vi "Start Node Drag.vi"(0 "FSM in":refnum<class "FSM.Graph.lvclass">, 5 "Node index":i32, 9 "Grid size":dbl, 11 "error in (no error)":errorcluster) -> (4 "FSM out":refnum<class "FSM.Graph.lvclass">, 8 "dragged nodes":string[](array[string]), 15 "error out":errorcluster)   [LabVIEW 2015, in "FSM.Graph.lvclass"]
uses:
  FSM.Graph.lvclass
  FSM.Graph.lvclass/FSM.Graph.ctl
  FSM.Node/FSM.Node.lvclass/FSM.Node.ctl
  FSM.Node/Read Name.vi
  FSM.Node/Read selected.vi
  FSM.Node/FSM.Node.lvclass
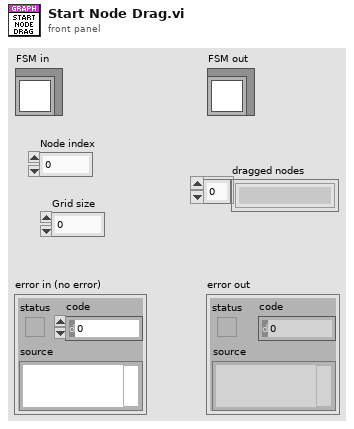
[diagram p1: front panel]
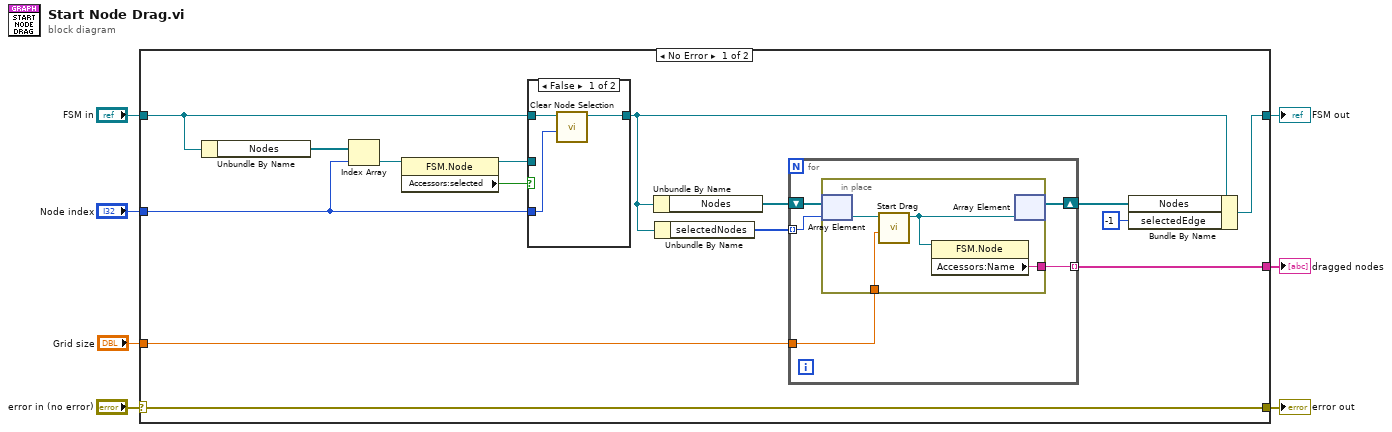
[diagram p0: block diagram]
diagram:
  n1 = case shown="No Error" "error in (no error)" {
    selector: "error in (no error)" -> [w22 w37]
    tunnel: [w22 w37] -> w6
    tunnel: [w12 w36] -> w4
    tunnel: "FSM in" -> [w16 w36]
    tunnel: "Node index" -> [w17 _]
    tunnel: "Grid size" -> [w10 _]
    tunnel: [w9 _] -> w1
    frame No Error {
      n2 = Unbundle By Name(w16) -> ("Nodes"=w21:refnum<class "FSM.Node.lvclass">[])
      n3 = Index Array(array=w21, index=w17) -> (element=w20:refnum<class "FSM.Node.lvclass">)
      n4 = property class="FSM.Node"(reference=w20) -> (reference out=w18:refnum<class "FSM.Node.lvclass">, "Accessors:selected"=w19:bool)  [unwired: 1 in, 1 out]
      n5 = case shown="False" w19 {
        tunnel: w18 -> [_ _]
        tunnel: w17 -> [w33 _]
        tunnel: w16 -> [w34 w35]
        tunnel: [w32 w35] -> w13
        frame False {
          n6 = call "Clear Node Selection.vi"("New selection"=w33, "FSM in"=w34) -> ("FSM out"=w32:refnum<class "FSM.Graph.lvclass">)  [unwired: 8 in, 1 out]
        }
        frame True {
        }
      }
      n7 = Unbundle By Name(w13) -> ("Nodes"=w14:refnum<class "FSM.Node.lvclass">[])
      n8 = Unbundle By Name(w13) -> ("selectedNodes"=w15:i32[])
      n9 = for {
        tunnel: w15 -> [w25] mode=indexing
        shift-right: [w24] -> w11
        shift-left: w14 -> [w26]
        tunnel: w10 -> [w27]
        tunnel: [w23] -> w9 mode=indexing
        n10 = in-place {
          in-place-border: w27 -> [w31]
          in-place-border: [w28] -> w23
          n11 = in-place-array #1(w26, w25) -> (w30:refnum<class "FSM.Node.lvclass">)
          n12 = call "Start Drag.vi"("Snap size"=w31, "FSM in"=w30) -> ("FSM out"=w29:refnum<class "FSM.Node.lvclass">)  [unwired: 8 in, 1 out]
          n13 = property class="FSM.Node"(reference=w29) -> ("Accessors:Name"=w28:string)  [unwired: 1 in, 2 out]
          n14 = in-place-array #1(w29) -> (w24:refnum<class "FSM.Node.lvclass">[])  [unwired: 1 out]
        }
      }
      n15 = Bundle By Name(cluster=w13, "Nodes"=w11, "selectedEdge"=-1) -> (w12:refnum<class "FSM.Graph.lvclass">)
    }
    frame Error {
    }
  }
  "error out" <- w6
  "FSM out" <- w4
  "dragged nodes" <- w1
